vi "JLINKARM Connect.vi"(8 "error in (no error)":errorcluster) -> (0 "error out":errorcluster, 3 "function return":i32)   [LabVIEW 2020, in "JLinkARM.lvlib"]
doc: "JLINKARMDLL_API int JLINKARM_Connect (void);"
uses:
  Lib/JLinkARM.lvlib
  JLinkARM.dll
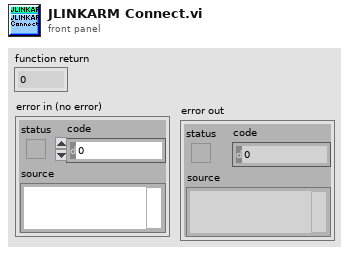
[diagram p1: front panel]
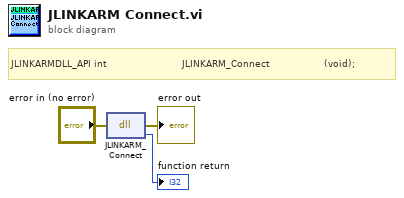
[diagram p0: block diagram]
diagram:
  # "JLINKARMDLL_API int                         JLINKARM_Connect                  (void);"
  n1 = dll-call lib="C:/Users/anybody/Desktop/JLinkARM.*" fn="JLINKARM_Connect"(error in="error in (no error)") -> (error out=→"error out":errorcluster, →"function return":i32)  [unwired: 2 in, 1 out]
